vi "Read DAQ FIFO.vi"(8 "error in (no error)":errorcluster, 9 "Timeout (ms)":i32, 10 "Data In":T1[](array[typedef]), 11 "CIF_NIChn_FIFO_DAQ in":refnum<class "CIF_NIChn_FIFO_DAQ_DVR.lvclass">) -> (0 "error out":errorcluster, 1 "timed out?":bool, 2 "Data Out":T1[](array[typedef]), 3 "CIF_NIChn_FIFO_DAQ out":refnum<class "CIF_NIChn_FIFO_DAQ_DVR.lvclass">, 4 "Header":T2)   [LabVIEW 2021, in "CIF_NIChn_FIFO_DAQ_DVR.lvclass"]
uses:
  CIF_NIChn_FIFO_DAQ_DVR.lvclass
  D:/dev/Packages/Channel_Manager/src/CIFChannels/CIFChannels.lvclass
  D:/dev/Packages/Channel_Manager/src/CIF_NIChn/FIFO_U8/CIF_NIChn_Fifo_U8.lvclass
  ChannelCommon/typedef/FIFO Header.ctl
  ChannelCommon/typedef/Datatype Waveform.ctl
  CIFChannels/CIFChannels.lvclass/CIFChannels.ctl
  FIFO_U8/CIF_NIChn_Fifo_U8.lvclass/CIF_NIChn_Fifo_U8.ctl
  CIF_NIChn_FIFO_DAQ_DVR.lvclass/CIF_NIChn_FIFO_DAQ_DVR.ctl
  <vilib>/CIF Foundation/CIF Utilities/Statistics/I64/Stats_I64_CIF_U.lvclass/Stats_I64_CIF_U.ctl
  SubVIs/DVR Unflatten.vi
  SubVIs/Unflatten.vi/4ab41953-a001-49d2-beab-55370b6c3c42.vi
  SubVIs/Unflatten.vi/7cd889b7-face-4678-a9e3-2692853b6930.vi
  CIFChannels/Utilities/Update Flatten Benchmark.vi
  CIFChannels/Accessors/Write FIFO Header.vi
  CIFChannels/Accessors/Write FIFO Timeout.vi
  FIFO_U8/Accessors/Read Payload.vi
  ChannelCommon/Utilities/Unflatten Header.vi
  ChannelCommon/Utilities/Add Error.vi
  <vilib>/CIF Foundation/CIF Utilities/DataTypes/Unflatten U64.vi
  <vilib>/CIF Foundation/CIF Utilities/Time/System Time/Get System Time.vi
  <vilib>/CIF Foundation/CIF Utilities/Statistics/I64/X1 minus X0.vi
  <vilib>/CIF Foundation/CIF Utilities/DataTypes/Unflatten I64.vi
  <vilib>/CIF Foundation/CIF Utilities/Errors/Append Error Location.vi
  <vilib>/CIF Foundation/CIF Utilities/Time/System Time/LabVIEW Time to TAI Time.vi
  <vilib>/CIF Foundation/CIF Utilities/Statistics/I64/X1 minus X0.vi/dfabcf33-0dbc-4041-80a5-3dc0c86d2989.vi
  <vilib>/CIF Foundation/CIF Utilities/Statistics/I64/X1 minus X0.vi/dfabcf33-0dbc-4041-80a5-3dc0c86d2989.vi/9eb60a9a-770f-4d2d-8b3f-8465c267ecc9.vi
  FIFO_U8/CIF_NIChn_Fifo_U8.lvclass
  D:/dev/Packages/Channel_Manager/src/CIF_NIChn/NIChn/CIF_NIChn.lvclass
  D:/dev/Packages/Channel_Manager/src/CIF_NIChn/FIFO_DAQ_DVR/CIF_NIChn_FIFO_DAQ_DVR.lvclass
  ChannelCommon/ChannelCommon.lvlib
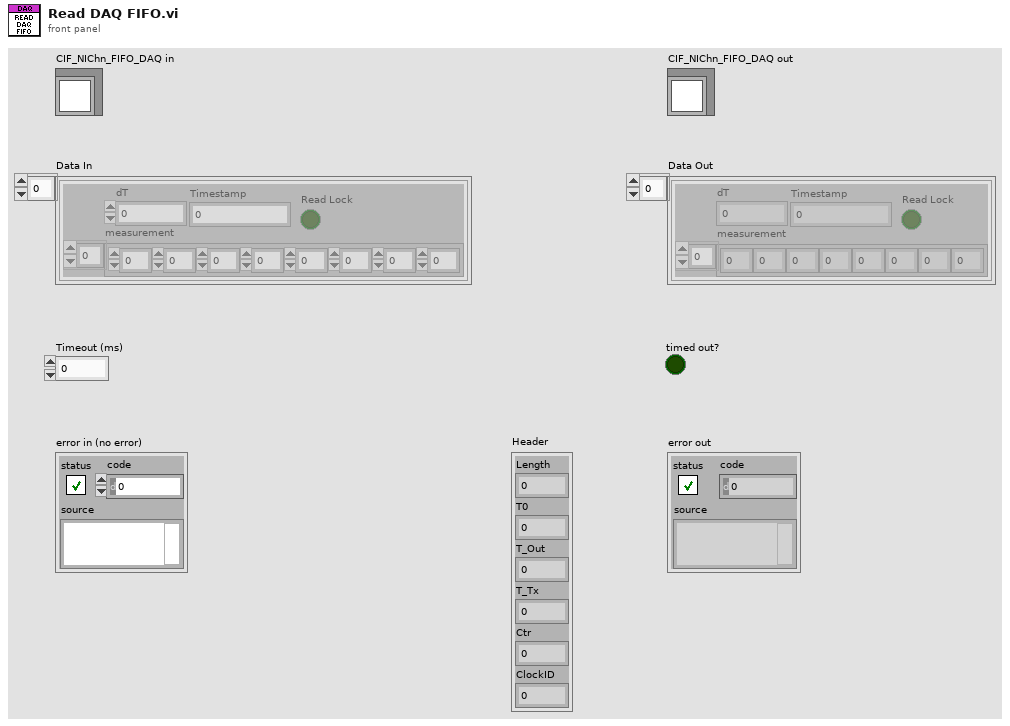
[diagram p1: front panel]
types:
  T1 = typedef "ChannelCommon.lvlib/Datatype Waveform.ctl" = cluster{"measurement":dbl[], "dT":dbl, "Timestamp":i64, "Read Lock":bool}
  T2 = typedef "ChannelCommon.lvlib/FIFO Header.ctl" = cluster{"Length":u64, "T0":i64, "T_Out":i64, "T_Tx":i64, "Ctr":u64, "ClockID":u8}
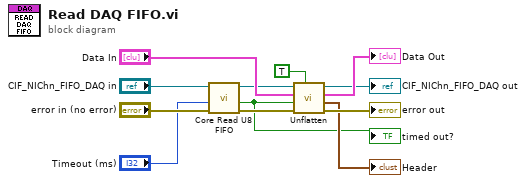
[diagram p0: block diagram]
diagram:
  n1 = call "Core Read U8 FIFO.vi"("error in (no error)"="error in (no error)", "Timeout (ms)"="Timeout (ms)", "CIFFIFO in"="CIF_NIChn_FIFO_DAQ in") -> ("error out"=w3:errorcluster, "timed out?"=w2:bool, "CIFFIFO out"=w4:refnum<class "CIF_NIChn_FIFO_DAQ_DVR.lvclass">)  [unwired: 6 in]
  "timed out?" <- w2
  n2 = call "Unflatten.vi"("Release Lock"=TRUE, "error in (no error)"=w3, "Timeout"=w2, "DAQ In"="Data In", "CIF_NIChn_FIFO_DAQ in"=w4) -> ("error out"=→"error out":errorcluster, "Header"=→"Header":T2, "DAQ Out"=→"Data Out":T1[], "CIF_NIChn_FIFO_DAQ out"=→"CIF_NIChn_FIFO_DAQ out":refnum<class "CIF_NIChn_FIFO_DAQ_DVR.lvclass">)  [unwired: 3 in]
